vi "Emi Cmd.vi"(0 "X-CAN en entrée":refnum<class "X-CAN.lvclass">, 1 "Num Image [1..32] :":u8=1 min=1 max=32 step=1, 2 "Page Haute :":bool, 3 "Type volet :":u16(ring) items=["Aucun", "Ouvrant gauche", "Ouvrant droite", "Ouvrant central", "Fermant gauche", "Fermant droite", "Fermant central"], 4 "Vitesse volet [1 .. 255] ms :":u8, 5 "entrée d'erreur (pas d'erreur)":errorcluster, 6 "Val luminosité :":u8, 7 "Periode clignottement":u8, 8 "Emission":bool, 9 "Periode affichage 2 images":u8, 10 "Commande à executer :":u16(ring) items=["Mise à jour Luminosité", "Appel Image", "Appel Image + Volet", "Affichage Page Basse", "Affichage Page Haute", "Mise à jour clignottement", "Affichage 2 images"]) -> (14 "X-CAN en sortie":refnum<class "X-CAN.lvclass">, 19 "sortie d'erreur":errorcluster)   [LabVIEW 2014]
uses:
  <vilib>/Stratom, Inc/X-CAN for myRIO (API)/X-CAN Class/X-CAN.lvclass
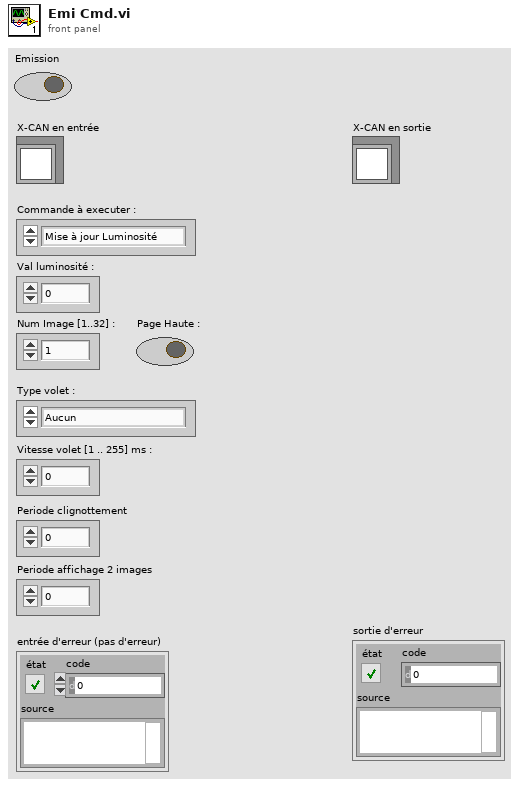
[diagram p1: front panel]
types:
  T1 = cluster{i32, bool, bool, u16[], "seconds since 1Jan1904":timestamp}
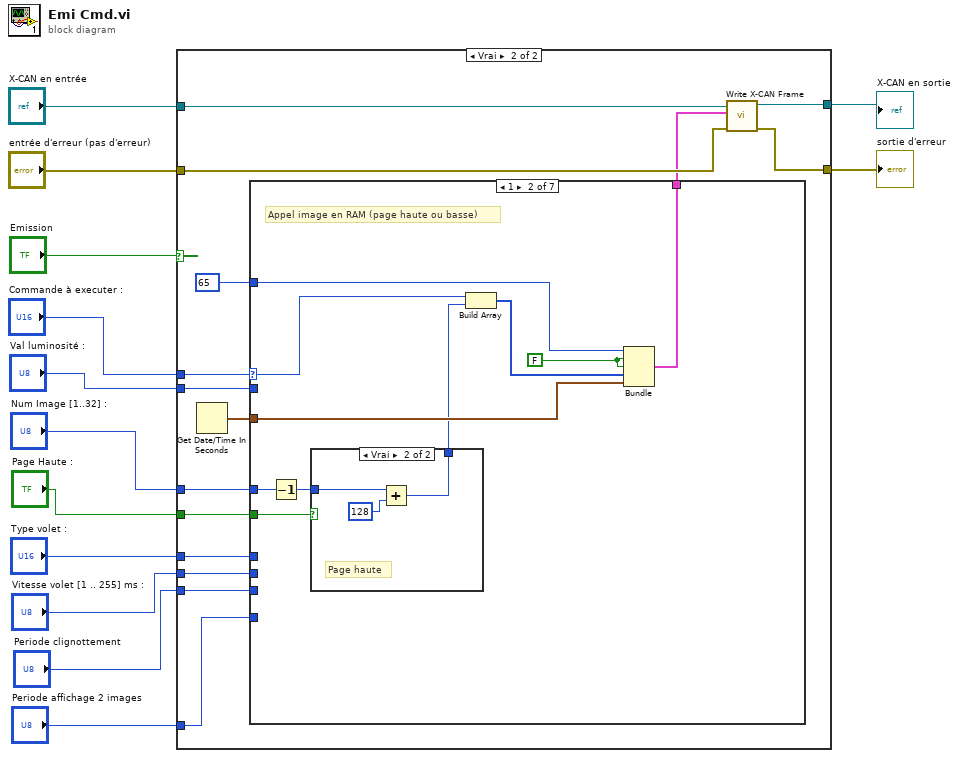
[diagram p0: block diagram]
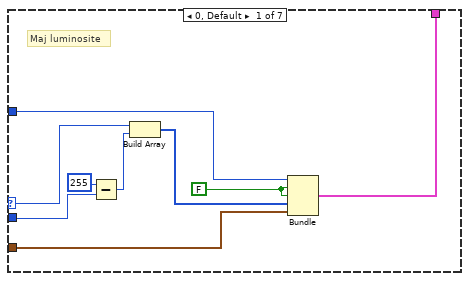
[diagram p3: hidden frame]
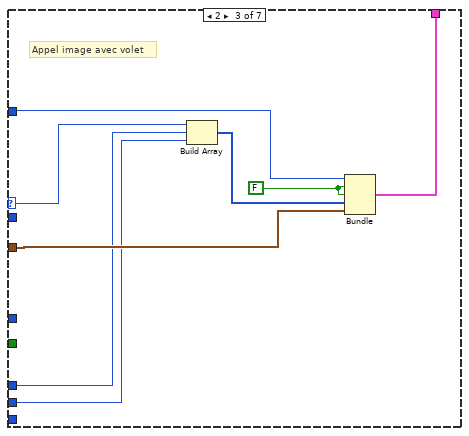
[diagram p5: hidden frame]
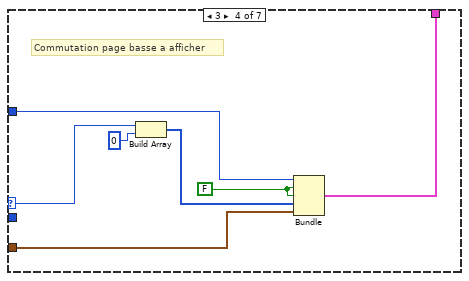
[diagram p6: hidden frame]
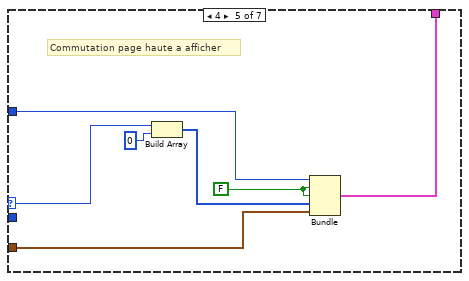
[diagram p7: hidden frame]
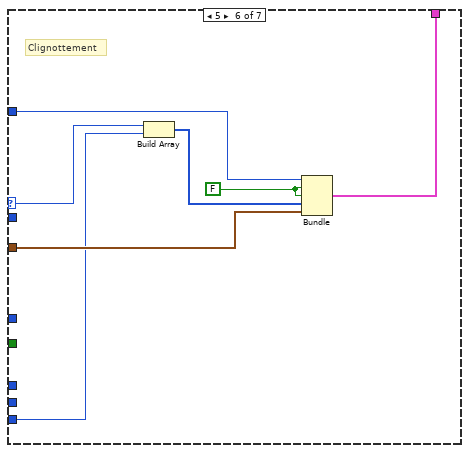
[diagram p8: hidden frame]
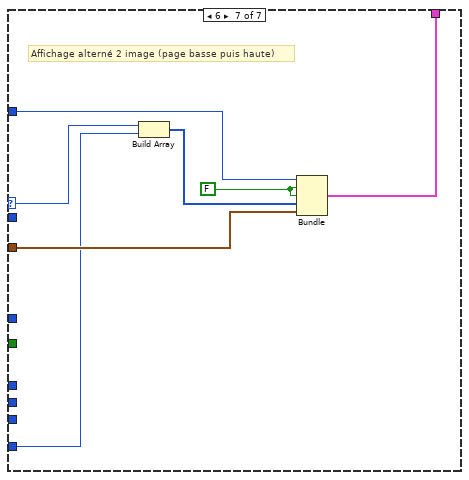
[diagram p9: hidden frame]
diagram:
  n1 = case shown="Vrai" "Emission" {
    tunnel: [w14 w30] -> w13
    tunnel: "entrée d'erreur (pas d'erreur)" -> [w14 w29]
    tunnel: [w15 w28] -> w11
    tunnel: "X-CAN en entrée" -> [w15 w27]
    tunnel: "Commande à executer :" -> [_ w26]
    tunnel: "Val luminosité :" -> [_ w22]
    tunnel: "Page Haute :" -> [_ w21]
    tunnel: "Num Image [1..32] :" -> [_ w20]
    tunnel: "Type volet :" -> [_ w19]
    tunnel: "Vitesse volet [1 .. 255] ms :" -> [_ w18]
    tunnel: "Periode clignottement" -> [_ w17]
    tunnel: "Periode affichage 2 images" -> [_ w16]
    frame False {
    }
    frame True {
      n2 = Get Date/Time In Seconds() -> (seconds since 1Jan1904=w25:timestamp)
      n3 = case shown="1" w26 {
        selector: w26 -> [w34 w45 w57 w64 w71 w77 w85]
        tunnel: w25 -> [w37 w46 w58 w65 w70 w79 w86]
        tunnel: 65 -> [w36 w47 w59 w66 w72 w80 w87]
        tunnel: [w35 w42 w54 w62 w69 w78 w83] -> w23
        tunnel: w22 -> [w32 _ _ _ _ _ _]
        tunnel: w21 -> [_ w44 _ _ _ _ _]
        tunnel: w20 -> [_ w41 _ _ _ _ _]
        tunnel: w19 -> [_ _ w56 _ _ _ _]
        tunnel: w18 -> [_ _ w55 _ _ _ _]
        tunnel: w17 -> [_ _ _ _ _ w76 _]
        tunnel: w16 -> [_ _ _ _ _ _ w84]
        frame 0, Default {
          w38 = FALSE
          # "Maj luminosite"
          n4 = Subtract(x=u8 255, y=w32) -> (x-y=w31:u8)
          n5 = Build Array(w34, w31) -> (w39:u16[])
          n6 = Bundle(w36, w38, w38, w39, "seconds since 1Jan1904"=w37) -> (w35:T1)  [unwired: 1 in]
        }
        frame 1 {
          w48 = FALSE
          # "Appel image en RAM (page haute ou basse)"
          n7 = Decrement(x=w41) -> (x-1=w40:u8)
          n8 = case shown="Vrai" w44 {
            tunnel: w40 -> [w50 w53]
            tunnel: [w50 w51] -> w43
            frame False {
              # "Page basse"
            }
            frame True {
              # "Page haute"
              n9 = Add(x=w53, y=u8 128) -> (x+y=w51:u8)
            }
          }
          n10 = Build Array(w45, w43) -> (w49:u16[])
          n11 = Bundle(w47, w48, w48, w49, "seconds since 1Jan1904"=w46) -> (w42:T1)  [unwired: 1 in]
        }
        frame 2 {
          w60 = FALSE
          # "Appel image avec volet"
          n12 = Build Array(w57, w56, w55) -> (w61:u16[])
          n13 = Bundle(w59, w60, w60, w61, "seconds since 1Jan1904"=w58) -> (w54:T1)  [unwired: 1 in]
        }
        frame 3 {
          w67 = FALSE
          # "Commutation page basse a afficher"
          n14 = Build Array(w64, u8 0) -> (w68:u16[])
          n15 = Bundle(w66, w67, w67, w68, "seconds since 1Jan1904"=w65) -> (w62:T1)  [unwired: 1 in]
        }
        frame 4 {
          w74 = FALSE
          # "Commutation page haute a afficher"
          n16 = Build Array(w71, u8 0) -> (w75:u16[])
          n17 = Bundle(w72, w74, w74, w75, "seconds since 1Jan1904"=w70) -> (w69:T1)  [unwired: 1 in]
        }
        frame 5 {
          w82 = FALSE
          # "Clignottement"
          n18 = Build Array(w77, w76) -> (w81:u16[])
          n19 = Bundle(w80, w82, w82, w81, "seconds since 1Jan1904"=w79) -> (w78:T1)  [unwired: 1 in]
        }
        frame 6 {
          w88 = FALSE
          # "Affichage alterné 2 image (page basse puis haute)"
          n20 = Build Array(w85, w84) -> (w89:u16[])
          n21 = Bundle(w87, w88, w88, w89, "seconds since 1Jan1904"=w86) -> (w83:T1)  [unwired: 1 in]
        }
      }
      n22 = call <vilib>:"Write X-CAN Frame.vi"("error in"=w29, "CAN Frame"=w23, "X-CAN Session in"=w27) -> ("error out"=w30:errorcluster, "X-CAN Session out"=w28:refnum<class "X-CAN.lvclass">)  [unwired: 7 in]
    }
  }
  "sortie d'erreur" <- w13
  "X-CAN en sortie" <- w11
